vi "ReadWrite.Data.Commit.vi"(8 "error in (no error)":errorcluster, 11 "Ref":T1) -> (0 "error out":errorcluster)   [LabVIEW 2023, in "Data Access Engine.lvlib" / "Data Access Engine.lvclass"]
uses:
  Data Access Engine.lvclass
  Access Type Classes/ReadWrite/ReadWrite.lvclass
  Access Type Classes/ReadWrite/ReadWrite.lvclass/ReadWrite.ctl
  Types/ReadWrite.DVR.ctl
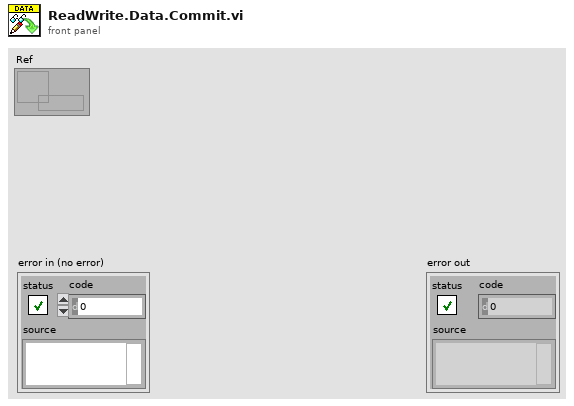
[diagram p1: front panel]
types:
  T1 = typedef "Data Access Engine.lvlib/Data Access Engine.lvclass/ReadWrite.DVR.ctl" = refnum<data-value>
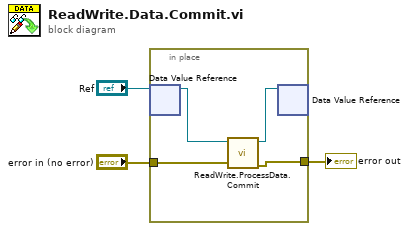
[diagram p0: block diagram]
diagram:
  n1 = in-place {
    in-place-border: "error in (no error)" -> [w5]
    in-place-border: [w4] -> w1
    n2 = in-place-dvr #1("Ref") -> (w7:refnum<class "ReadWrite.lvclass">)  [unwired: 1 out]
    n3 = call "ReadWrite.ProcessData.Commit.vi"("error in (no error)"=w5, "ReadWrite in"=w7) -> ("error out"=w4:errorcluster, "ReadWrite out"=w6:refnum<class "ReadWrite.lvclass">)  [unwired: 8 in]
    n4 = in-place-dvr #1(w6) -> ()  [unwired: 2 out]
  }
  "error out" <- w1
